vi "confirm stop moving.vi"(11 "moving?":bool) -> (3 "Boolean":bool)   [LabVIEW 2018]
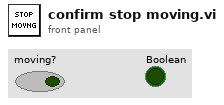
[diagram p1: front panel]
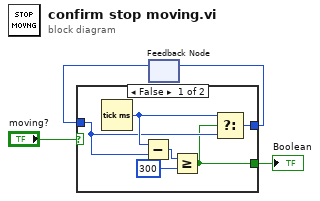
[diagram p0: block diagram]
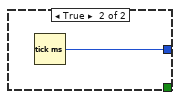
[diagram p2: hidden frame]
diagram:
  n1 = feedback #1() -> (w2:u32)  [unwired: 1 in]
  n2 = case shown="False" "moving?" {
    tunnel: [w7 w11] -> w3
    tunnel: w2 -> [w6 _]
    tunnel: [w5 _] -> w1
    frame False {
      n3 = Tick Count (ms)() -> (millisecond timer value=w8:u32)
      n4 = Subtract(x=w8, y=w6) -> (x-y=w10:u32)
      n5 = Greater Or Equal?(x=w10, y=u32 300) -> (x >= y?=w5:bool)
      n6 = Select(t=w8, s=w5, f=w6) -> (s? t:f=w7:u32)
    }
    frame True {
      n7 = Tick Count (ms)() -> (millisecond timer value=w11:u32)
    }
  }
  "Boolean" <- w1
  n8 = feedback-in #1(w3) -> ()
